vi "Untitled 3.vi"() -> ()   [LabVIEW 2014]
panel:
  out "Waveform Chart":dbl(graph)
  out "Waveform Graph":dbl[](graph)
  out "Array":dbl[](array[numeric])
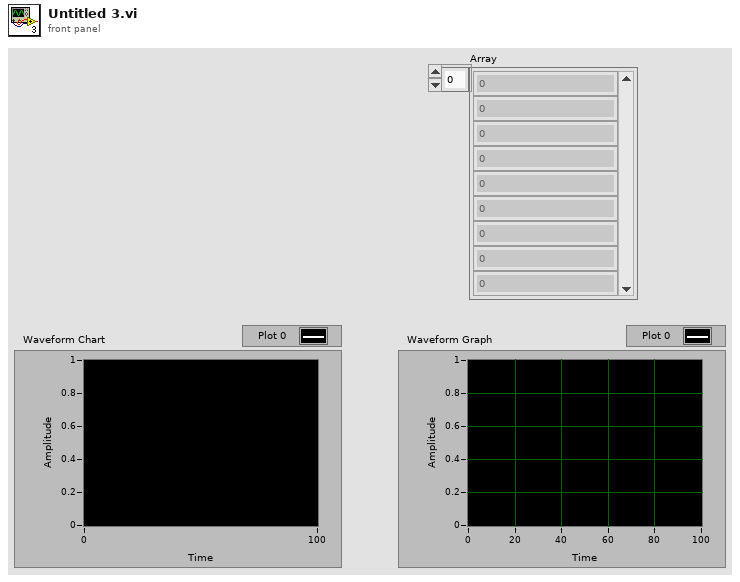
[diagram p1: front panel]
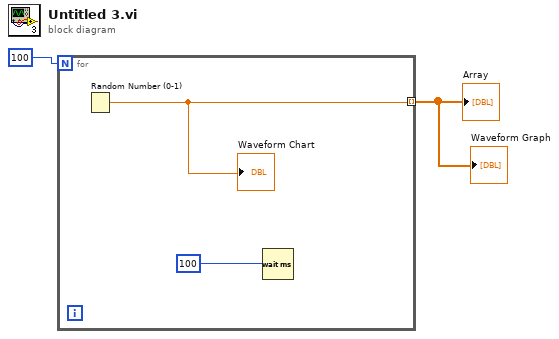
[diagram p0: block diagram]
diagram:
  n1 = for {
    N: 100 -> [_]
    tunnel: [w4] -> w1 mode=indexing
    n2 = Random Number (0-1)() -> (number: 0 to 1=w4:dbl)
    "Waveform Chart" <- w4
    n3 = Wait (ms)(milliseconds to wait=100) -> ()  [unwired: 1 out]
  }
  "Array" <- w1
  "Waveform Graph" <- w1
